vi "Read Title.vi"(8 "error in (no error)":errorcluster, 11 "SampleDescriptionHolder in":refnum<class "MetaDataObj.lvclass">) -> (0 "error out":errorcluster, 2 "Title":string, 3 "SampleDescriptionHolder out":refnum<class "MetaDataObj.lvclass">)   [LabVIEW 2016, in "MetaDataObj.lvclass"]
uses:
  <resource>/dialog/NewProjectWizard/MetaDataObj/MetaDataObj.lvclass
  <resource>/dialog/NewProjectWizard/MetaDataObj/MetaDataObj.lvclass/MetaDataObj.ctl
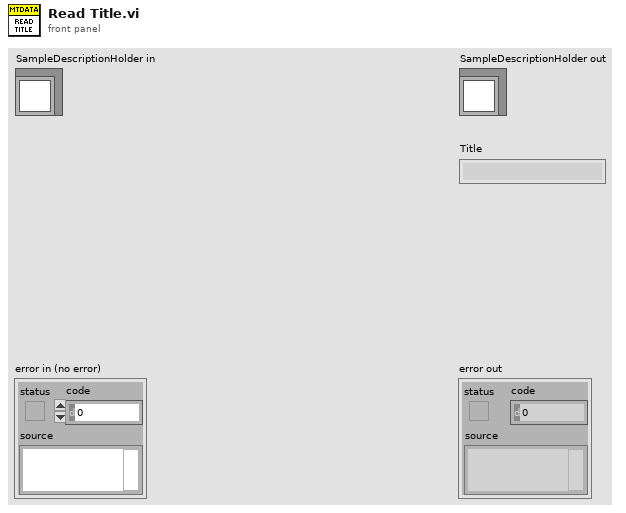
[diagram p1: front panel]
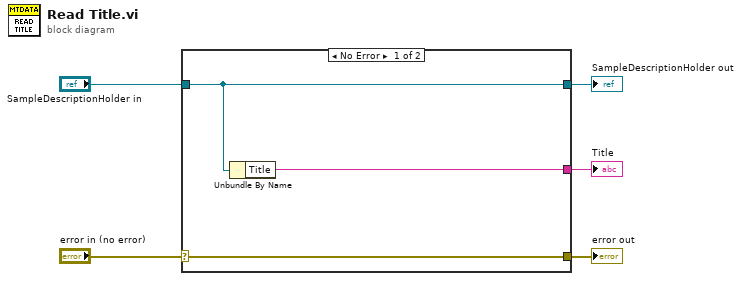
[diagram p0: block diagram]
diagram:
  n1 = case shown="No Error" "error in (no error)" {
    selector: "error in (no error)" -> [w8 w9]
    tunnel: [w8 w9] -> w4
    tunnel: [w7 w10] -> w2
    tunnel: "SampleDescriptionHolder in" -> [w7 w10]
    tunnel: [w6 _] -> w1
    frame No Error {
      n2 = Unbundle By Name(w7) -> ("Title"=w6:string)
    }
    frame Error {
    }
  }
  "error out" <- w4
  "SampleDescriptionHolder out" <- w2
  "Title" <- w1
